vi "Devantech SRF08 Sonar.vi"() -> ()   [LabVIEW 2025]
doc: "This example shows how to use the SRF08 Ultrasonic Range Finder via the I2C bus. It can display the distance from the sensor in inches or centimeters.\n\nThis example expects a USB cable connected from your development PC to the Type B USB Jack (next to the power input) on the roboRIO."
uses:
  <vilib>/Rock Robotics/SystemInterfaces/i2clib/i2c_bus.ctl
  <vilib>/Rock Robotics/WPI/Ultrasonic/WPI_SonarSRF08DeviceAddress.ctl
  <vilib>/Rock Robotics/WPI/Ultrasonic/WPI_SonarSRF08_I2C_Open.vi
  <vilib>/Rock Robotics/WPI/Ultrasonic/WPI_SonarSRF08_I2C_GetRange.vi
  <vilib>/Rock Robotics/WPI/Ultrasonic/WPI_SonarSRF08_I2C_Close.vi
panel:
  in  "Range Units":u8(ring)=80 items=["Inches"=80, "Centimeters"=81, "Microseconds"=82]
  in  "Device Address":T1=224 items=["Dev 0"=224, "Dev 1"=226, "Dev 2"=228, "Dev 3"=230, "Dev 4"=232, "Dev 5"=234, "Dev 6"=236, "Dev 7"=238, "Dev 8"=240, "Dev 9"=242, "Dev 10"=244, "Dev 11"=246, "Dev 12"=248, "Dev 13"=250, "Dev 14"=252, "Dev 15"=254]
  in  "I2C Bus":T2
  out "Light Sensor":u8
  out "Distance":u16
  in  "stop":bool
  # "Set these inputs before running."
  # "This can be set while running."
  # "Output information."
  # "This shows wiring for the SRF08 ultrasonic range finder.\nNote the I2C header provides 3.3V, so this sensor gets its 5V power from the 5V rail - in this case DIO-0."
  # "SRF08\nGnd (black wire)------\nPower (red wire)------\nSCL (yellow wire)-----\nSDA (white wire)------"
  # "roboRIO\nI2C  \nDIO0   V\nI2C   SCL\nI2C   SDA"
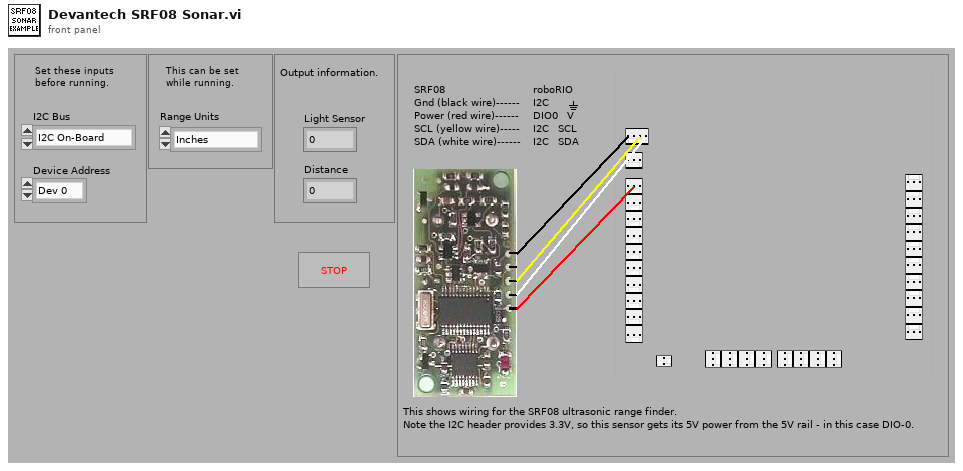
[diagram p1: front panel]
types:
  T1 = typedef "WPI_SonarSRF08DeviceAddress.ctl" = u8
  T2 = typedef "i2c_bus.ctl" = enum16{"I2C On-Board", "I2C MXP", "Invalid"}
  T3 = typedef "WPI_SonarSRF08_I2C_DeviceRef.ctl" = cluster{"I2CDevRef":T4}
  T4 = typedef "WPI_I2CDevRef.ctl" = cluster{"DevStatus":errorcluster, "Device Address":u8, "Handle":i32, "I2C Bus":T2}
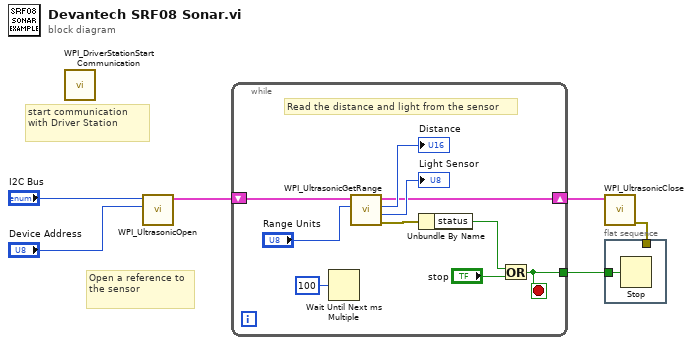
[diagram p0: block diagram]
diagram:
  # "start communication with Driver Station"
  # "Open a reference to the sensor"
  n1 = call <vilib>:"WPI_DriverStationStart Communication.vi"() -> ()  [unwired: 3 in, 9 out]
  n2 = call-poly <vilib>:"WPI_UltrasonicOpen.vi"("Device Address"="Device Address", "I2C Bus"="I2C Bus") -> ("SonarSRF08_I2C_DevRef"=w3:T3)  [unwired: 8 in, 1 out]
  n3 = while {
    tunnel: [w14] -> w6
    shift-right: [w7] -> w2
    shift-left: w3 -> [w12]
    stop <- w14 stop-if-true
    # "Read the distance and light from the sensor"
    n4 = Wait Until Next ms Multiple(millisecond multiple=u32 100 ("milliseconds to wait")) -> ()  [unwired: 1 out]
    n5 = call-poly <vilib>:"WPI_UltrasonicGetRange.vi"("Range Units"="Range Units", "SonarSRF08_I2C_DevRef"=w12) -> ("error out"=w10:errorcluster, "Light Sensor"=→"Light Sensor":u8, "Distance"=→"Distance":u16, "SonarSRF08_I2C_DevRef"=w7:T3)  [unwired: 6 in]
    n6 = Unbundle By Name(w10) -> ("status"=w16:bool)
    n7 = Or(x=w16, y="stop") -> (x .or. y?=w14:bool)
  }
  n8 = call-poly <vilib>:"WPI_UltrasonicClose.vi"("SonarSRF08_I2C_DevRef"=w2) -> ("error out"=w1:errorcluster)  [unwired: 10 in]
  n9 = flat-sequence {
    tunnel: w6 -> [w17]
    tunnel: w1 -> [_]
    frame #0 {
      n10 = Stop(stop? (T)=w17) -> ()
    }
  }
